vi "Read Timeout.vi"(8 "error in (no error)":errorcluster, 11 "OnChange_Boolean in":refnum<class "OnChangeNotifier_DBL.lvclass">) -> (0 "error out":errorcluster, 2 "Timeout":bool, 3 "OnChange_Boolean out":refnum<class "OnChangeNotifier_DBL.lvclass">)   [LabVIEW 2021, in "OnChangeNotifier_DBL.lvclass"]
uses:
  OnChangeNotifier_DBL.lvclass
  OnChangeNotifier_DBL.lvclass/OnChangeNotifier_DBL.ctl
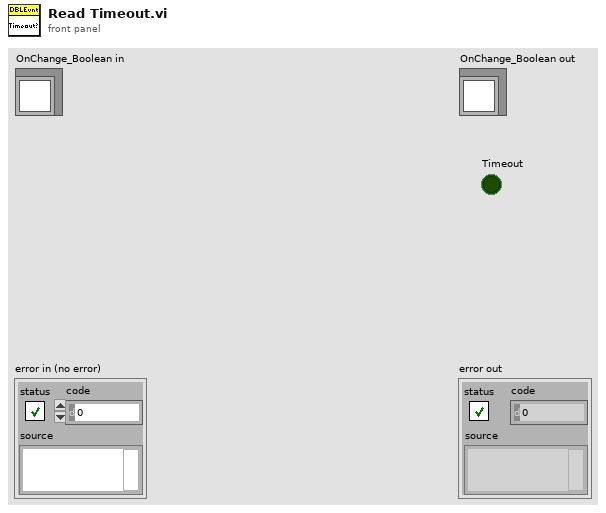
[diagram p1: front panel]
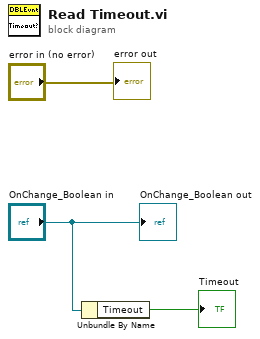
[diagram p0: block diagram]
diagram:
  n1 = Unbundle By Name("OnChange_Boolean in") -> ("Timeout"=→"Timeout":bool)
  "error out" <- "error in (no error)"
  "OnChange_Boolean out" <- "OnChange_Boolean in"
